vi "Perform Action.vi"(8 "error in":errorcluster, 10 "Input":variant, 11 "DI DAQmx CFG in":refnum<class "DI DAQmx Meas Freq CFG.lvclass">) -> (0 "error out":errorcluster, 2 "Output":variant, 3 "DI DAQmx CFG out":refnum<class "DI DAQmx Meas Freq CFG.lvclass">)   [LabVIEW 2023, in "DI DAQmx Meas Freq CFG.lvclass"]
uses:
  DI DAQmx Meas Freq CFG.lvclass
  DAQmx/DAQmx Base CFG/DAQmx Base CFG.lvclass
  <vilib>/DAQmx/read.llb/DAQmx Read (Digital 1D Bool 1Chan 1Samp).vi
panel:
  out "data 2":cluster{"Channel":string}
  out "data":bool[](array[boolean])
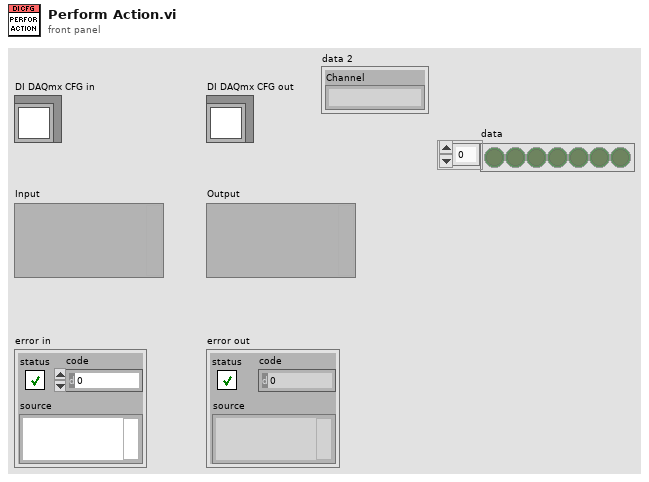
[diagram p1: front panel]
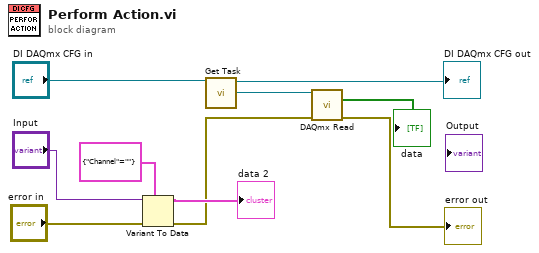
[diagram p0: block diagram]
diagram:
  n1 = Variant To Data(error in="error in", type=cluster{"Channel":string} {"Channel"=""}, Variant="Input") -> (data=→"data 2":cluster{"Channel":string}, error out=w1:errorcluster)
  n2 = call "Get Task.vi"("DAQmx Base CFG in"="DI DAQmx CFG in") -> ("Task"=w7:refnum<k21>, "DAQmx Base CFG out"=→"DI DAQmx CFG out":refnum<class "DI DAQmx Meas Freq CFG.lvclass">)  [unwired: 9 in]
  n3 = call-poly <vilib>:"DAQmx Read.vi"("task/channels in"=w7, "error in"=w1) -> ("data"=→"data":bool[], "error out"=→"error out":errorcluster)  [unwired: 11 in, 1 out]
